vi "LV_Asana_UI_Mockup.vi"() -> ()   [LabVIEW 2016]
panel:
  out "spreadsheet string":string
  in  "device name: SA0XXXX.YYYYMMDD":string
  in  "project":u16(ring) items=["Quasi-1D chiral proteins", "CZO/STO nanowriting", "Alex Hamilton", "CoO2 nano-sheets", "CoO2 nanoflakes", "TaAs Hall Bar", "Ken Burch 2D Materials on LAOSTO", "Bawendi lead halide nano crystals", "SrIrO3-doped LAO/STO", "Superconductivity in Ti4O7 and \\gamma-Ti3O5 films"]
  in  "get user names":bool
  in  "Stop":bool
  in  "user":u16(ring) items=["Shan Hao", "Megan Briggeman", "Aditi Nethwewala", "Dengyue Yang", "Erin Sutton", "Lu Chen", "Yun-Yi Pai", "Yuhe Tang", "Jessica Montone", "Qing Guo", "Joe Albro", "Jianan Li", "Jeremy Levy", "Patrick Irvin"]
  # "1. press to get user names"
  # "2. choose a user"
  # "3. choose a project"
  # "4. choose or type in a\ndevice"
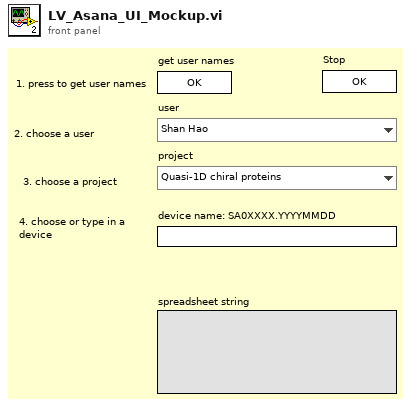
[diagram p1: front panel]
types:
  T1 = enum32{"invalid app kind", "Development System", "Run Time System", "Student Edition", "Embedded LabVIEW", "Evaluation", "Custom"}
  T2 = enum32{"Invalid", "Standard", "Closed", "Hidden", "Minimized", "Maximized"}
  T3 = cluster{"Core":cluster{"Current VI Reference":refnum<vi>, "Close Panel on Exit?":bool}, "Your Boolean data":bool, "user string":string, "research project string":string, "device string":string}
  T4 = cluster{"Current VI Reference":refnum<vi>, "Close Panel on Exit?":bool}
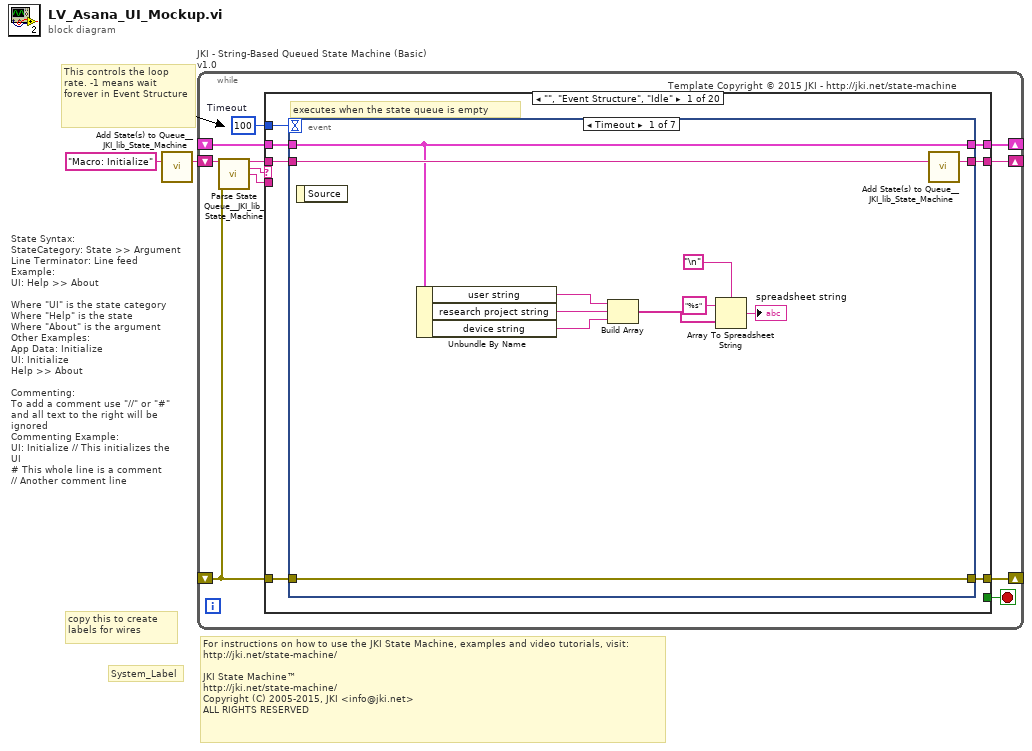
[diagram p0: block diagram]
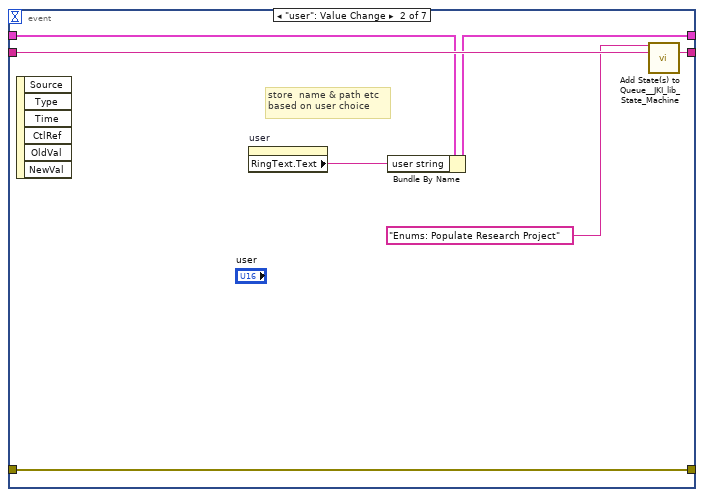
[diagram p2: hidden frame]
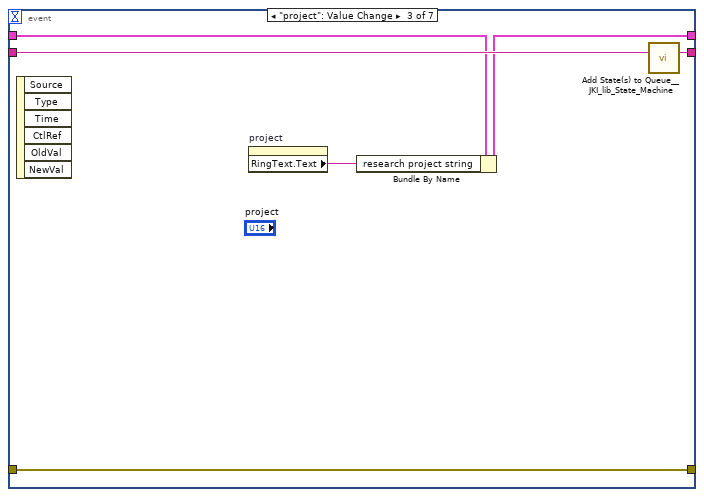
[diagram p3: hidden frame]
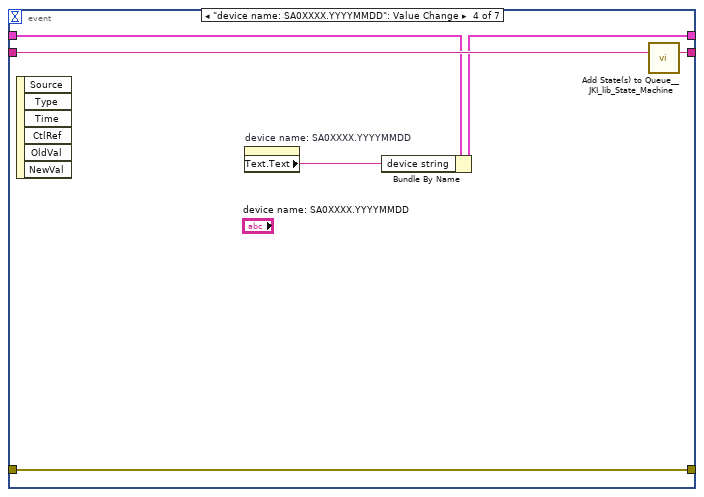
[diagram p4: hidden frame]
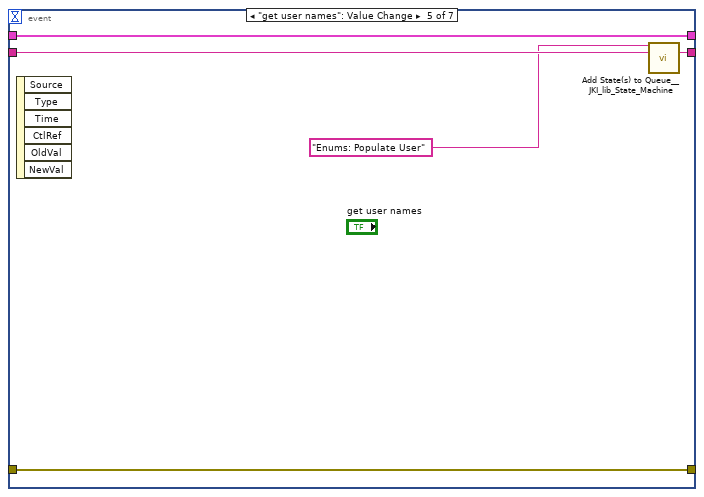
[diagram p5: hidden frame]
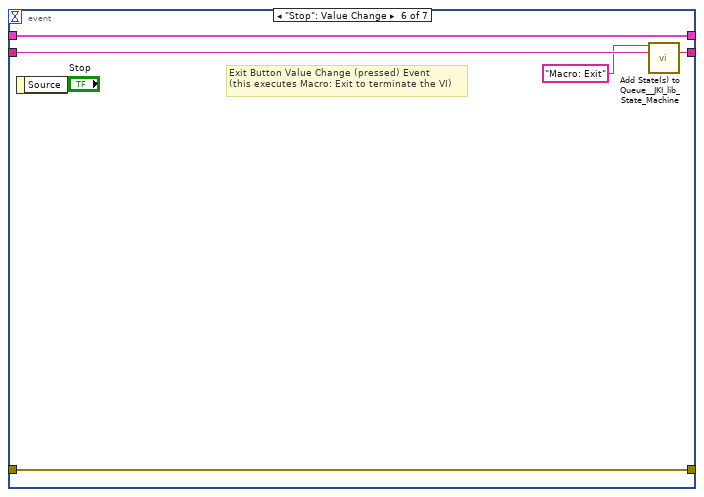
[diagram p6: hidden frame]
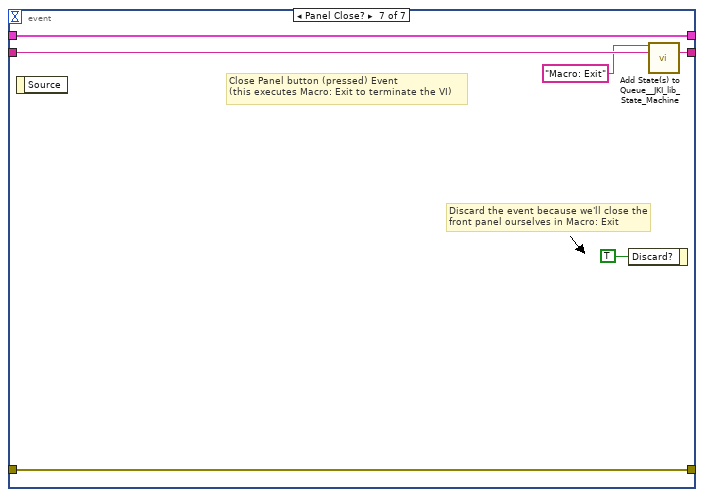
[diagram p7: hidden frame]
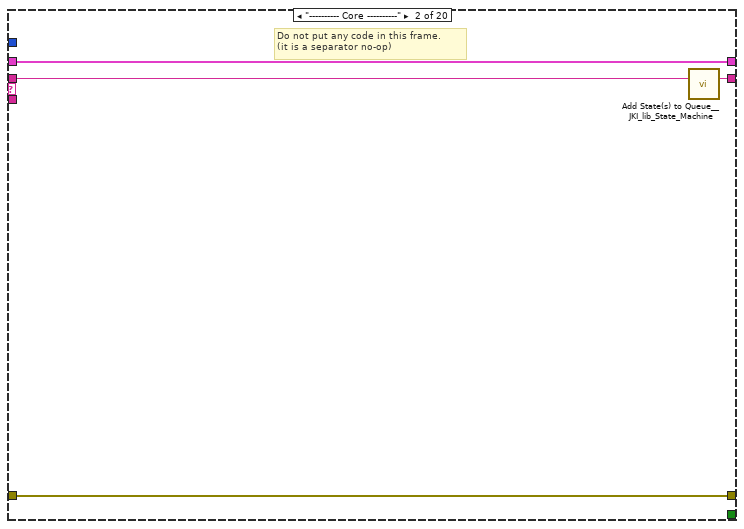
[diagram p8: hidden frame]
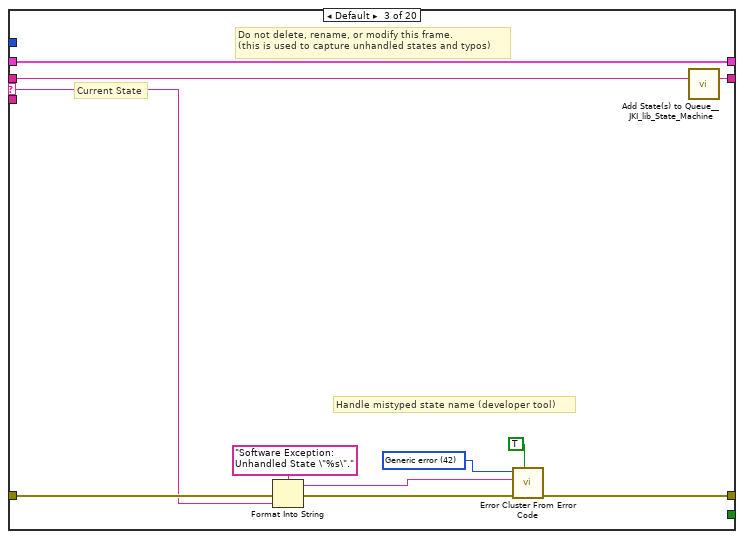
[diagram p9: hidden frame]
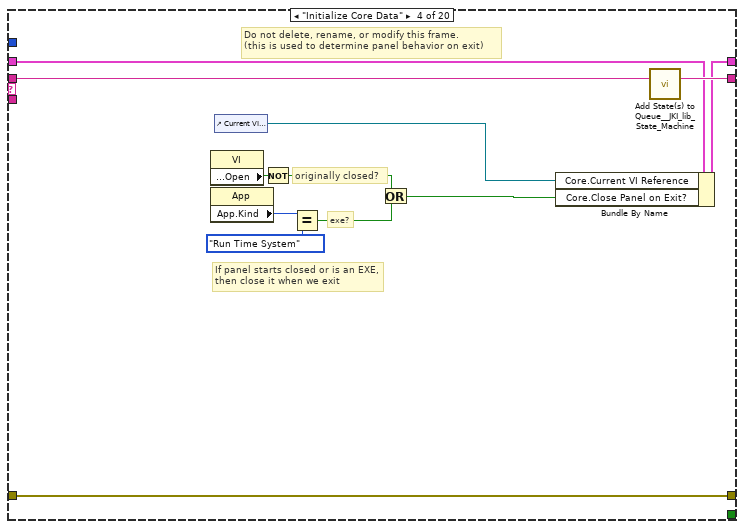
[diagram p10: hidden frame]
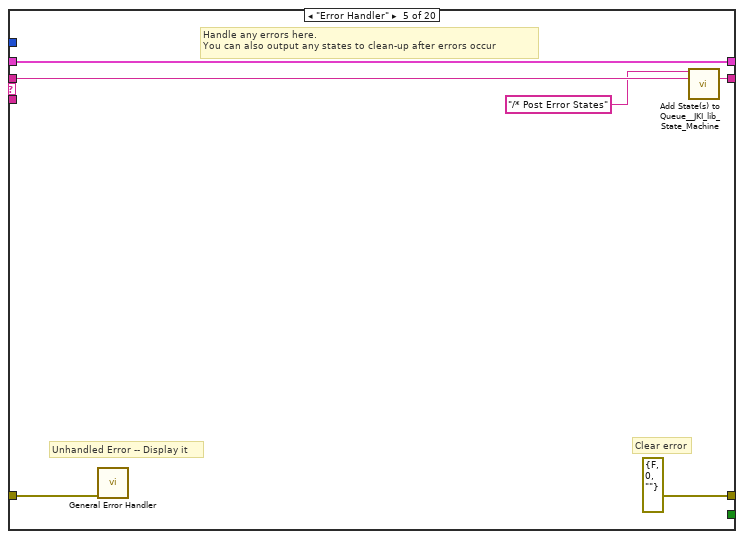
[diagram p11: hidden frame]
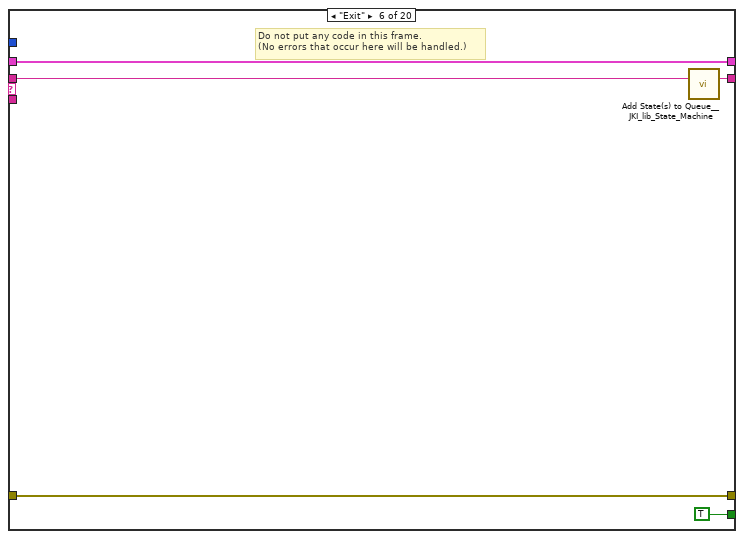
[diagram p12: hidden frame]
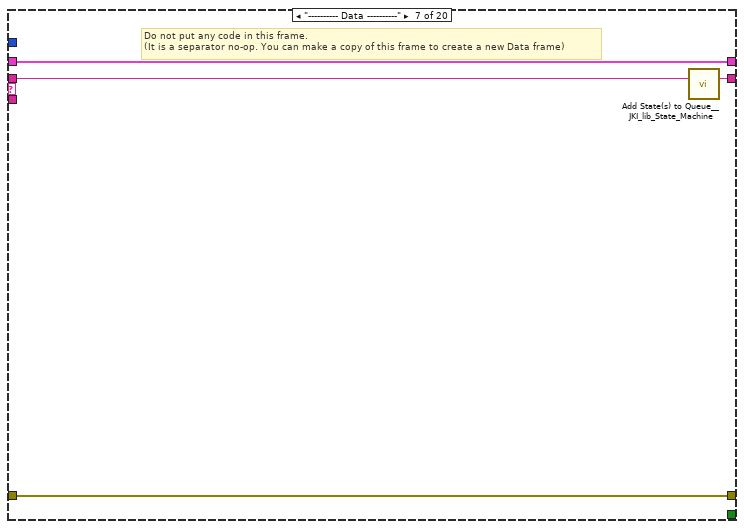
[diagram p13: hidden frame]
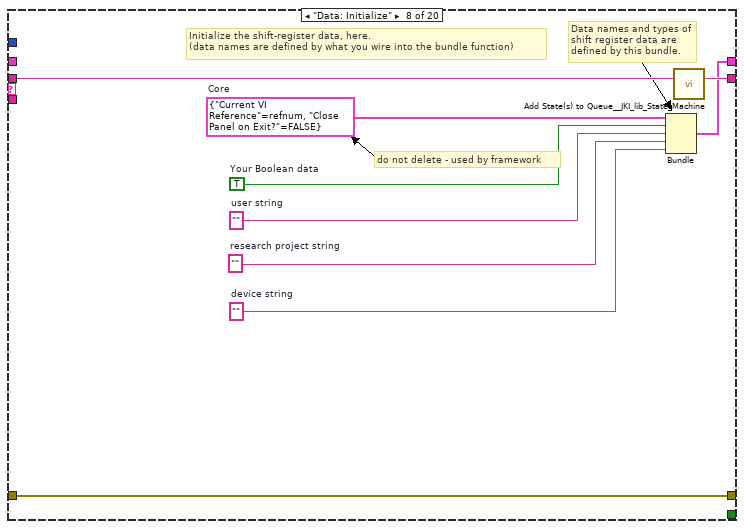
[diagram p14: hidden frame]
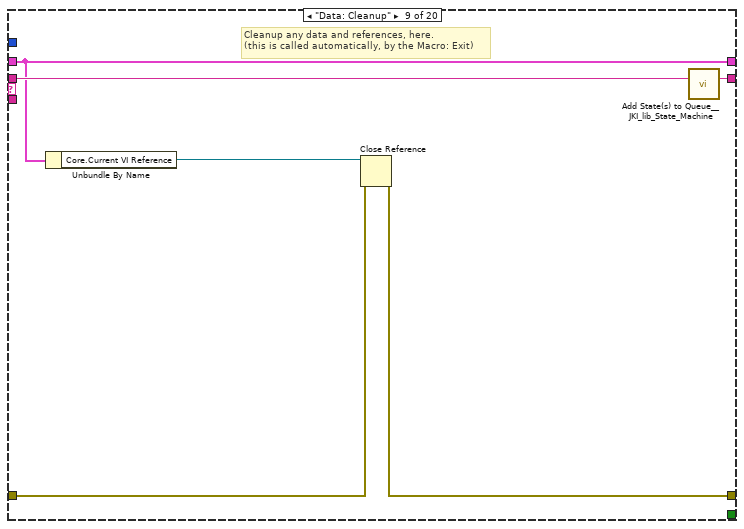
[diagram p15: hidden frame]
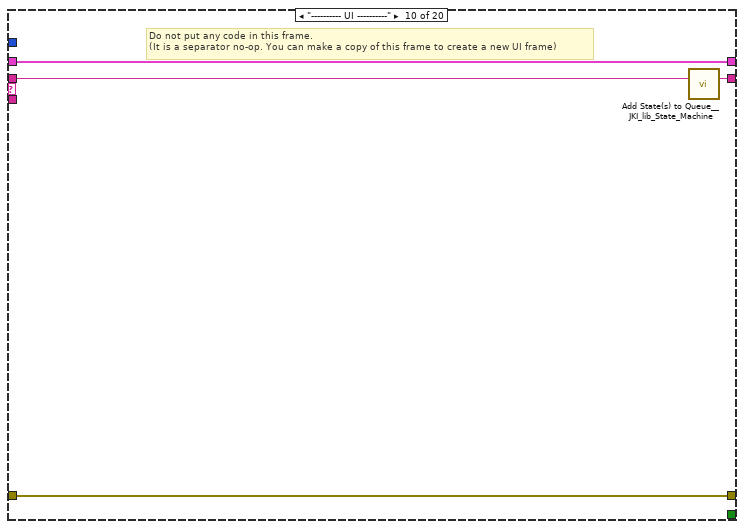
[diagram p16: hidden frame]
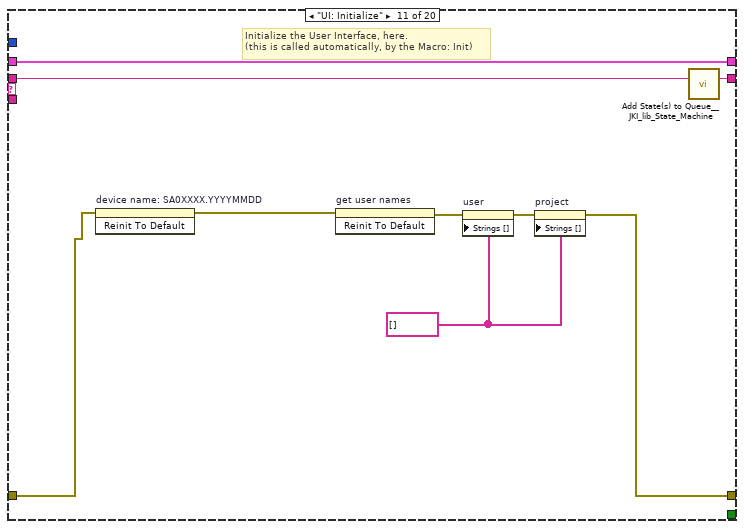
[diagram p17: hidden frame]
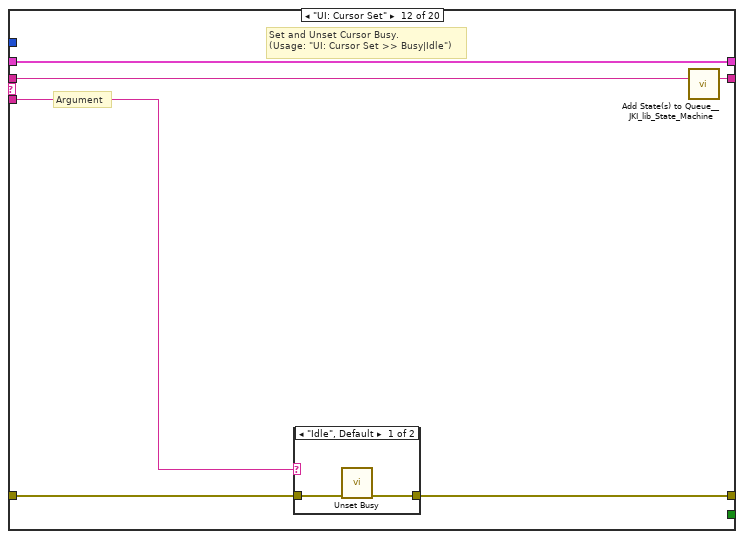
[diagram p18: hidden frame]
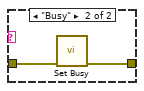
[diagram p19: hidden frame]
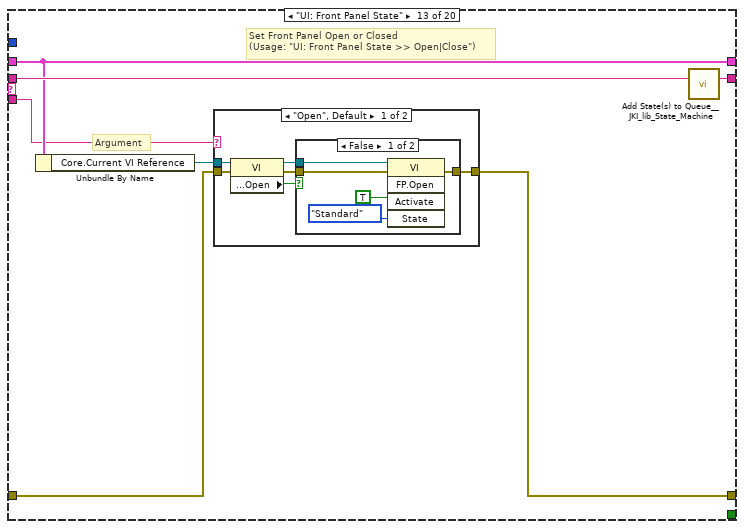
[diagram p20: hidden frame]
diagram:
  # "For instructions on how to use the JKI State Machine, examples and video tutorials, visit:\nhttp://jki.net/state-machine/\n\nJKI State Machine™\nhttp://jki.net/state-machine/\nCopyright (C) 2005-2015, JKI <info@jki.net>\nALL RIGHTS RESERVED"
  # "State Syntax:\nStateCategory: State >> Argument\nLine Terminator: Line feed\nExample:\nUI: Help >> About\n\nWhere \"UI\" is the state category\nWhere \"Help\" is the state\nWhere \"About\" is the argument\nOther Examples:\nApp Data: Initialize\nUI: Initialize\nHelp >> About\n\nCommenting:\nTo add a comment use \"//\" or \"#\" and all text to the right will be ignored\nCommenting Example:\nUI: Initialize // This initializes the UI\n# This whole line is a comment\n// Another comment line"
  # "copy this to create labels for wires"
  # "This controls the loop rate. -1 means wait forever in Event Structure"
  # "System_Label"
  n1 = call <vilib>:"Add State(s) to Queue__JKI_lib_State_Machine.vi"("State(s) in (\"\")"="Macro: Initialize") -> ("States Out"=w2:string)  [unwired: 14 in]
  n2 = while "JKI - String-Based Queued State Machine (Basic) v1.0" {
    shift-right: [w6] -> _
    shift-left: _ -> [w5]
    shift-right: [w9] -> _
    shift-left: _ -> [w3]
    shift-right: [w8] -> _
    shift-left: w2 -> [w10]
    stop <- w7 stop-if-true
    w4 = 100  # Timeout
    # "Template Copyright © 2015 JKI - http://jki.net/state-machine"
    n3 = call <vilib>:"Parse State Queue__JKI_lib_State_Machine.vi"("State Queue"=w10, "Error In (no error)"=w3) -> ("Remaining States"=w12:string, "Current State"=w13:string, "Arguments"=w11:string)  [unwired: 11 in]
    n4 = case shown="\"\", \"Event Structure\", \"Idle\"" w13 {
      selector: w13 -> [_ _ w71 _ _ _ _ _ _ _ _ _ _ _ _ _ _ _ _ _]
      tunnel: w12 -> [w20 w70 w75 w93 w99 w104 w108 w117 w123 w127 w136 w142 w153 w179 w184 w194 w198 w203 w212 w217]
      tunnel: w11 -> [_ _ _ _ _ _ _ _ _ _ _ w137 w147 _ _ _ _ _ _ _]
      tunnel: w5 -> [w18 w67 w73 w84 w96 w102 w105 _ w118 w124 w134 w140 w149 w176 w181 w191 w195 w200 w209 w214]
      tunnel: [w17 w68 w77 w90 errorcluster {"status"=FALSE, "code"=0, "source"=""} ("error out") w101 w106 w114 w119 w125 w128 w138 w150 w177 w182 w192 w196 w201 w210 w215] -> w9
      tunnel: w3 -> [w16 w68 w76 w90 w95 w101 w106 w114 w120 w125 w133 w139 w151 w177 w182 w192 w196 w201 w210 w215]
      tunnel: [w19 w69 w74 w92 w98 w103 w107 w116 w122 w126 w135 w141 w152 w178 w183 w193 w197 w202 w211 w216] -> w8
      tunnel: [_ _ _ _ _ TRUE _ _ _ _ _ _ _ _ _ _ _ _ _ _] -> w7
      tunnel: [w15 w67 w73 w91 w96 w102 w105 w115 w118 w124 w134 w140 w149 w176 w181 w191 w195 w200 w209 w214] -> w6
      tunnel: w4 -> [w14 _ _ _ _ _ _ _ _ _ _ _ _ _ _ _ _ _ _ _]
      frame "", "Event Structure", "Idle" {
        # "executes when the state queue is empty"
        n5 = event shown="[0] Timeout" {
          selector: _ -> [_ _ _ _ _ _ _]
          dyn-events: _ -> [_ _ _ _ _ _ _]
          timeout: w14 -> [_ _ _ _ _ _ _]
          tunnel: w20 -> [w31 w38 w44 w50 w55 w60 w66]
          tunnel: [w30 w37 w43 w49 w54 w59 w65] -> w19
          tunnel: w18 -> [w28 w35 w41 w47 w52 w57 w63]
          tunnel: [w29 w36 w42 w48 w53 w58 w64] -> w17
          tunnel: w16 -> [w29 w36 w42 w48 w53 w58 w64]
          tunnel: [w28 w34 w40 w46 w52 w57 w63] -> w15
          event Timeout {
            n6 = event-data() -> ()  [unwired: 1 in, 1 out]
            n7 = Unbundle By Name(w28) -> ("user string"=w26:string, "research project string"=w27:string, "device string"=w25:string)
            n8 = Build Array(w26, w27, w25) -> (w24:string[])
            n9 = Array To Spreadsheet String(delimiter (Tab)="\n", array=w24, 3:"%s" ("format string")) -> (spreadsheet string=→"spreadsheet string":string)
            n10 = call <vilib>:"Add State(s) to Queue__JKI_lib_State_Machine.vi"("State(s) in (\"\")"=w31) -> ("States Out"=w30:string)  [unwired: 14 in]
          }
          event "user": Value Change {
            # "store  name & path etc\nbased on user choice"
            n11 = event-data() -> ()  [unwired: 1 in, 6 out]
            n12 = property on="user" class="Ring (strict)"() -> ("RingText.Text"=w33:string)  [unwired: 2 in, 2 out]
            n13 = Bundle By Name(cluster=w35, "user string"=w33) -> (w34:T3)
            n14 = call <vilib>:"Add State(s) to Queue__JKI_lib_State_Machine.vi"("State(s) in Front (\"\")"="Enums: Populate Research Project" ("State(s) in Front (\"\")"), "State(s) in (\"\")"=w38) -> ("States Out"=w37:string)  [unwired: 13 in]
          }
          event "project": Value Change {
            n15 = event-data() -> ()  [unwired: 1 in, 6 out]
            n16 = property on="project" class="Ring (strict)"() -> ("RingText.Text"=w39:string)  [unwired: 2 in, 2 out]
            n17 = Bundle By Name(cluster=w41, "research project string"=w39) -> (w40:T3)
            n18 = call <vilib>:"Add State(s) to Queue__JKI_lib_State_Machine.vi"("State(s) in (\"\")"=w44) -> ("States Out"=w43:string)  [unwired: 14 in]
          }
          event "device name: SA0XXXX.YYYYMMDD": Value Change {
            n19 = event-data() -> ()  [unwired: 1 in, 6 out]
            n20 = property on="device name: SA0XXXX.YYYYMMDD" class="Str"() -> ("Text.Text"=w45:string)  [unwired: 2 in, 2 out]
            n21 = Bundle By Name(cluster=w47, "device string"=w45) -> (w46:T3)
            n22 = call <vilib>:"Add State(s) to Queue__JKI_lib_State_Machine.vi"("State(s) in (\"\")"=w50) -> ("States Out"=w49:string)  [unwired: 14 in]
          }
          event "get user names": Value Change {
            n23 = event-data() -> ()  [unwired: 1 in, 6 out]
            n24 = call <vilib>:"Add State(s) to Queue__JKI_lib_State_Machine.vi"("State(s) in Front (\"\")"="Enums: Populate User" ("State(s) in Front (\"\")"), "State(s) in (\"\")"=w55) -> ("States Out"=w54:string)  [unwired: 13 in]
          }
          event "Stop": Value Change {
            # "Exit Button Value Change (pressed) Event\n(this executes Macro: Exit to terminate the VI)"
            n25 = event-data() -> ()  [unwired: 1 in, 1 out]
            n26 = call <vilib>:"Add State(s) to Queue__JKI_lib_State_Machine.vi"("State(s) in Front (\"\")"="Macro: Exit", "State(s) in (\"\")"=w60) -> ("States Out"=w59:string)  [unwired: 13 in]
          }
          event Panel Close? {
            # "Discard the event because we'll close the front panel ourselves in Macro: Exit"
            # "Close Panel button (pressed) Event\n(this executes Macro: Exit to terminate the VI)"
            n27 = event-data() -> ()  [unwired: 1 in, 1 out]
            n28 = event-data("Discard?"=TRUE) -> ()  [unwired: 1 in, 1 out]
            n29 = call <vilib>:"Add State(s) to Queue__JKI_lib_State_Machine.vi"("State(s) in Front (\"\")"="Macro: Exit", "State(s) in (\"\")"=w66) -> ("States Out"=w65:string)  [unwired: 13 in]
          }
        }
      }
      frame "---------- Core ----------" {
        # "Do not put any code in this frame.\n(it is a separator no-op)"
        n30 = call <vilib>:"Add State(s) to Queue__JKI_lib_State_Machine.vi"("State(s) in (\"\")"=w70) -> ("States Out"=w69:string)  [unwired: 14 in]
      }
      frame Default {
        w80 = 42 items=["No error", "Argument error", "Memory is full", "Out of zone", "End of file", "File already open", "Generic file I/O error", "File not found", "File permission error", "Disk is full", "Duplicate path", "Too many files open", "System feature not enabled", "Resource file not found", "Cannot add resource", "Resource not found", "Image not found", "Image memory error", "Pen does not exist", "Config type invalid", "Config token not found", "Config parse error", "Config memory error", "Bad external code format", "Bad external code offset", "External code not present", "Null window", "Destroy window error", "Null menu", "Print aborted", "Bad print record", "Print driver error", "Windows error during printing", "Memory error during printing", "Print dialog error", "Generic print error", "Invalid device refnum", "Device not found", "Device parameter error", "Device unit error", "Cannot open device", "Device call aborted", "Generic error", "Cancelled by user", "Object ID too low", "Object ID too high", "Object not in heap", "Unknown heap", "Unknown object (invalid DefProc)", "Unknown object (DefProc not in table)", "Message out of range", "Invalid (null) method", "Unknown message", "Manager call not supported", "Bad address", "Network operation in progress", "Network operation timed out", "Connection is busy", "Network attribute not supported", "Network error", "Address in use", "System out of memory", "Connection aborted", "Connection refused", "Not connected", "Already connected", "Connection closed", "Initialization error (interapplication manager)", "Bad occurrence", "Wait on unbound occurrence handler", "Occurrence queue overflow", "Datalog type conflict", "Unused", "Unrecognized type (interapplication manager)", "Memory corrupt", "Failed to make temporary DLL", "Old CIN version", "Drag socket not found", "Failed to load drop-object", "Failed to register OLE object", "Failed to release OLE object", "Format specifier type mismatch", "Unknown format specifier", "Too few format specifiers", "Too many format specifiers", "Scan failed", "Newer CIN version", "Error converting to variant", "Runtime menu error", "Password tampered", "Variant attribute not found", "Incompatible variant data type", "Event data is not available", "Event Store is not present", "Occurrence is not found", "Event Queue is not created", "Event info is not available", "Refnum passed is NULL", "Error retrieving Class GUID", "Error retrieving CoClass GUID", "Error retrieving TypeLib GUID.", "Bad built application magic bytes.", "Specific driver is different from the specific driver associated with the Logical Name.", "There is no session opened to the class driver.", "Max Error", "MAX - Error with config objects", "MAX - Error loading configuration", "MAX - Group not supported"]
        # "Current State"
        # "Do not delete, rename, or modify this frame.\n(this is used to capture unhandled states and typos)"
        # "Handle mistyped state name (developer tool)"
        n31 = Format Into String(format string="Software Exception: Unhandled State \"%s\"." ("message"), error in=w76, w71) -> (resulting string=w79:string, error out=w78:errorcluster)  [unwired: 1 in]
        n32 = call <vilib>:"Error Cluster From Error Code.vi"("show call chain? (False)"=TRUE, "error in (no error)"=w78, "error message (\"\")"=w79, "error code (0)"=w80) -> ("error out"=w77:errorcluster)  [unwired: 5 in]
        n33 = call <vilib>:"Add State(s) to Queue__JKI_lib_State_Machine.vi"("State(s) in (\"\")"=w75) -> ("States Out"=w74:string)  [unwired: 14 in]
      }
      frame "Initialize Core Data" {
        # "Do not delete, rename, or modify this frame.\n(this is used to determine panel behavior on exit)"
        # "originally closed?"
        # "exe?"
        # "If panel starts closed or is an EXE, then close it when we exit"
        n34 = property class="VI"() -> ("Front Panel.Open"=w89:bool)  [unwired: 2 in, 2 out]
        n35 = property class="App"() -> ("App.Kind"=w88:T1)  [unwired: 2 in, 2 out]
        n36 = control-ref of="Current VI Reference"() -> (w82:refnum<vi>)
        n37 = Not(x=w89) -> (.not. x?=w86:bool)
        n38 = Equal?(x=w88, y=T1."Run Time System" ("Application:Kind")) -> (x = y?=w85:bool)
        n39 = Or(x=w86, y=w85) -> (x .or. y?=w83:bool)
        n40 = Bundle By Name(cluster=w84, "Core.Current VI Reference"=w82, "Core.Close Panel on Exit?"=w83) -> (w91:T3)
        n41 = call <vilib>:"Add State(s) to Queue__JKI_lib_State_Machine.vi"("State(s) in (\"\")"=w93) -> ("States Out"=w92:string)  [unwired: 14 in]
      }
      frame "Error Handler" {
        # "Unhandled Error -- Display it"
        # "Handle any errors here.\nYou can also output any states to clean-up after errors occur"
        # "Clear error"
        n42 = call <vilib>:"General Error Handler.vi"("error in (no error)"=w95) -> ()  [unwired: 10 in, 5 out]
        n43 = call <vilib>:"Add State(s) to Queue__JKI_lib_State_Machine.vi"("State(s) in Front (\"\")"="/* Post Error States", "State(s) in (\"\")"=w99) -> ("States Out"=w98:string)  [unwired: 13 in]
      }
      frame "Exit" {
        # "Do not put any code in this frame.\n(No errors that occur here will be handled.)"
        n44 = call <vilib>:"Add State(s) to Queue__JKI_lib_State_Machine.vi"("State(s) in (\"\")"=w104) -> ("States Out"=w103:string)  [unwired: 14 in]
      }
      frame "---------- Data ----------" {
        # "Do not put any code in this frame.\n(It is a separator no-op. You can make a copy of this frame to create a new Data frame)"
        n45 = call <vilib>:"Add State(s) to Queue__JKI_lib_State_Machine.vi"("State(s) in (\"\")"=w108) -> ("States Out"=w107:string)  [unwired: 14 in]
      }
      frame "Data: Initialize" {
        w109 = ""  # device string
        w110 = ""  # research project string
        w111 = T4 {"Current VI Reference"=refnum, "Close Panel on Exit?"=FALSE}  # Core
        w113 = TRUE  # Your Boolean data
        w112 = ""  # user string
        # "do not delete - used by framework"
        # "Data names and types of shift register data are defined by this bundle."
        # "Initialize the shift-register data, here.\n(data names are defined by what you wire into the bundle function)"
        n46 = Bundle("Core"=w111, "Your Boolean data"=w113, "user string"=w112, "research project string"=w110, "device string"=w109) -> (w115:T3)  [unwired: 1 in]
        n47 = call <vilib>:"Add State(s) to Queue__JKI_lib_State_Machine.vi"("State(s) in (\"\")"=w117) -> ("States Out"=w116:string)  [unwired: 14 in]
      }
      frame "Data: Cleanup" {
        # "Cleanup any data and references, here.\n(this is called automatically, by the Macro: Exit)"
        n48 = Unbundle By Name(w118) -> ("Core.Current VI Reference"=w121:refnum<vi>)
        n49 = Close Reference(reference=w121, error in (no error)=w120) -> (error out=w119:errorcluster)
        n50 = call <vilib>:"Add State(s) to Queue__JKI_lib_State_Machine.vi"("State(s) in (\"\")"=w123) -> ("States Out"=w122:string)  [unwired: 14 in]
      }
      frame "---------- UI ----------" {
        # "Do not put any code in this frame.\n(It is a separator no-op. You can make a copy of this frame to create a new UI frame)"
        n51 = call <vilib>:"Add State(s) to Queue__JKI_lib_State_Machine.vi"("State(s) in (\"\")"=w127) -> ("States Out"=w126:string)  [unwired: 14 in]
      }
      frame "UI: Initialize" {
        w129 = string[] [] ("Strings []")
        # "Initialize the User Interface, here.\n(this is called automatically, by the Macro: Init)"
        n52 = invoke on="device name: SA0XXXX.YYYYMMDD" class="Str" method="Reinit To Default"(error in=w133) -> (error out=w132:errorcluster)  [unwired: 2 in, 2 out]
        n53 = invoke on="get user names" class="Bool" method="Reinit To Default"(error in=w132) -> (error out=w130:errorcluster)  [unwired: 2 in, 2 out]
        n54 = property on="user" class="Ring (strict)"(error in=w130, "Strings []"=w129) -> (error out=w131:errorcluster)  [unwired: 1 in, 1 out]
        n55 = property on="project" class="Ring (strict)"(error in=w131, "Strings []"=w129) -> (error out=w128:errorcluster)  [unwired: 1 in, 1 out]
        n56 = call <vilib>:"Add State(s) to Queue__JKI_lib_State_Machine.vi"("State(s) in (\"\")"=w136) -> ("States Out"=w135:string)  [unwired: 14 in]
      }
      frame "UI: Cursor Set" {
        # "Argument"
        # "Set and Unset Cursor Busy.\n(Usage: \"UI: Cursor Set >> Busy|Idle\")"
        n57 = case shown="\"Idle\", Default" w137 {
          tunnel: w139 -> [w144 w146]
          tunnel: [w143 w145] -> w138
          frame "Idle", Default {
            n58 = call <vilib>:"Unset Busy.vi"("error in (no error)"=w144) -> ("error out"=w143:errorcluster)  [unwired: 10 in]
          }
          frame "Busy" {
            n59 = call <vilib>:"Set Busy.vi"("error in (no error)"=w146) -> ("error out"=w145:errorcluster)  [unwired: 9 in, 1 out]
          }
        }
        n60 = call <vilib>:"Add State(s) to Queue__JKI_lib_State_Machine.vi"("State(s) in (\"\")"=w142) -> ("States Out"=w141:string)  [unwired: 14 in]
      }
      frame "UI: Front Panel State" {
        # "Argument"
        # "Set Front Panel Open or Closed\n(Usage: \"UI: Front Panel State >> Open|Close\")"
        n61 = Unbundle By Name(w149) -> ("Core.Current VI Reference"=w148:refnum<vi>)
        n62 = case shown="\"Open\", Default" w147 {
          tunnel: w151 -> [w157 w170]
          tunnel: [w159 w171] -> w150
          tunnel: w148 -> [w158 w168]
          frame "Open", Default {
            n63 = property class="VI"(reference=w158, error in=w157) -> (reference out=w155:refnum<vi>, error out=w156:errorcluster, "Front Panel.Open"=w154:bool)
            n64 = case shown="False" w154 {
              tunnel: [w162 w165] -> w159
              tunnel: w156 -> [w161 w165]
              tunnel: w155 -> [w160 _]
              frame False {
                n65 = invoke class="VI" method="FP.Open"(reference=w160, error in=w161, "Activate"=TRUE, "State"=T2."Standard") -> (error out=w162:errorcluster)  [unwired: 1 in, 4 out]
              }
              frame True {
              }
            }
          }
          frame "Close" {
            n66 = property class="VI"(reference=w168, error in=w170) -> (reference out=w167:refnum<vi>, error out=w169:errorcluster, "Front Panel.Open"=w166:bool)
            n67 = case shown="True" w166 {
              tunnel: [w172 w175] -> w171
              tunnel: w169 -> [w172 w174]
              tunnel: w167 -> [_ w173]
              frame False {
              }
              frame True {
                n68 = invoke class="VI" method="FP.Close"(reference=w173, error in=w174) -> (error out=w175:errorcluster)  [unwired: 1 in, 2 out]
              }
            }
          }
        }
        n69 = call <vilib>:"Add State(s) to Queue__JKI_lib_State_Machine.vi"("State(s) in (\"\")"=w153) -> ("States Out"=w152:string)  [unwired: 14 in]
      }
      frame "---------- Macro ----------" {
        # "Do not put any code in this frame.\n(It is a separator no-op. You can make a copy of this frame to create a new Macro frame)"
        n70 = call <vilib>:"Add State(s) to Queue__JKI_lib_State_Machine.vi"("State(s) in (\"\")"=w179) -> ("States Out"=w178:string)  [unwired: 14 in]
      }
      frame "Macro: Initialize" {
        w180 = "Data: Initialize\nInitialize Core Data\nUI: Initialize\nUI: Front Panel State >> Open"  # Data: Initialize Initialize Core Data UI: Initialize UI: Front Panel State >> Open
        # "Initialization Macro\n(This is called once, when the VI starts)"
        n71 = call <vilib>:"Add State(s) to Queue__JKI_lib_State_Machine.vi"("State(s) in Front (\"\")"=w180, "State(s) in (\"\")"=w184) -> ("States Out"=w183:string)  [unwired: 13 in]
      }
      frame "Macro: Exit" {
        # "Exit Macro\n(This is called once, when the VI exits)"
        n72 = Unbundle By Name(w191) -> ("Core.Close Panel on Exit?"=w190:bool)
        n73 = Select(t="UI: Front Panel State >> Close", s=w190, f="") -> (s? t:f=w187:string)
        n74 = call <vilib>:"Add State(s) to Queue__JKI_lib_State_Machine.vi"("State(s) in (\"\")"=w187, "State(s) at Back (\"\")"="Data: Cleanup\nExit") -> ("States Out"=w185:string)  [unwired: 13 in]
        n75 = call <vilib>:"Add State(s) to Queue__JKI_lib_State_Machine.vi"("State(s) in Front (\"\")"=w185, "State(s) in (\"\")"=w194) -> ("States Out"=w193:string)  [unwired: 13 in]
      }
      frame "---------- Enums ----------" {
        # "Template Separator\n(You can make a copy of, or modify, this frame)"
        n76 = call <vilib>:"Add State(s) to Queue__JKI_lib_State_Machine.vi"("State(s) in (\"\")"=w198) -> ("States Out"=w197:string)  [unwired: 14 in]
      }
      frame "Enums: Populate User" {
        # "Your code here.\n(You can make a copy of, or modify, this frame)"
        n77 = flat-sequence {
          tunnel: [w204] -> w199
          frame #0 {
            # "this code represents call to asana asking for users"
            n78 = Spreadsheet String To Array(delimiter (Tab)="\n", format string="%s", spreadsheet string="Shan Hao\nMegan Briggeman\nAditi Nethwewala\nDengyue Yang\nErin Sutton\nLu Chen\nYun-Yi Pai\nYuhe Tang\nJessica Montone\nQing Guo\nJoe Albro\nJianan Li\nJeremy Levy\nPatrick Irvin", array type (2D Dbl)=string[] []) -> (array=w204:string[])
          }
        }
        n79 = property on="user" class="Ring (strict)"("Strings []"=w199) -> ()  [unwired: 2 in, 2 out]
        n80 = call <vilib>:"Add State(s) to Queue__JKI_lib_State_Machine.vi"("State(s) in (\"\")"=w203) -> ("States Out"=w202:string)  [unwired: 14 in]
      }
      frame "Enums: Populate Sample" {
        # "Your code here.\n(You can make a copy of, or modify, this frame)"
        n81 = call <vilib>:"Add State(s) to Queue__JKI_lib_State_Machine.vi"("State(s) in (\"\")"=w212) -> ("States Out"=w211:string)  [unwired: 14 in]
      }
      frame "Enums: Populate Research Project" {
        # "Template Separator\n(You can make a copy of, or modify, this frame)"
        n82 = flat-sequence {
          tunnel: [w218] -> w213
          frame #0 {
            # "this code represents call to asana asking for research project names"
            n83 = Spreadsheet String To Array(delimiter (Tab)="\n", format string="%s", spreadsheet string="Quasi-1D chiral proteins\nCZO/STO nanowriting\nAlex Hamilton\nCoO2 nano-sheets\nCoO2 nanoflakes\nTaAs Hall Bar\nKen Burch 2D Materials on LAOSTO\nBawendi lead halide nano crystals\nSrIrO3-doped LAO/STO\nSuperconductivity in Ti4O7 and \\gamma-Ti3O5 films", array type (2D Dbl)=string[] []) -> (array=w218:string[])
          }
        }
        n84 = property on="project" class="Ring (strict)"("Strings []"=w213) -> ()  [unwired: 2 in, 2 out]
        n85 = call <vilib>:"Add State(s) to Queue__JKI_lib_State_Machine.vi"("State(s) in (\"\")"=w217) -> ("States Out"=w216:string)  [unwired: 14 in]
      }
    }
  }
